vi "Set SG Path.vi"(0 "Path in":refnum<class "SA Path.lvclass">, 5 "Cal point in":T1, 11 "error in":errorcluster) -> (4 "Path out":refnum<class "SA Path.lvclass">, 6 "Cal point out":T1, 8 "Source Gain":dbl, 10 "Digital Gain":dbl, 15 "error out":errorcluster)   [LabVIEW 2023, in "RFFixtureCharact.PXI.lvlib" / "SA Path.lvclass"]
uses:
  SA Path.lvclass
  Public/Base Classes/Scalar/Scalar Path/Type Definitions/Cal Point.ctl
  <vilib>/addons/_RFCalAndCharactDatabase/NI_RFCalAndCharact_Database_API.lvlibp/Characterization/Controls/Type.ctl
  Public/Base Classes/Scalar/SA Abstract Path/SA Abstract Path.lvclass/SA Abstract Path.ctl
  Public/Base Classes/Scalar/SA Abstract Path/Properties/Read Cal Tone Pin.vi
  <instrlib>/niRFSG/niRFSG.llb/niRFSG Create De-embedding S-parameter Table (array).vi
  Public/Base Classes/Scalar/SA Path/SA Path.lvclass
  <vilib>/addons/_RFCalAndCharactDatabase/NI_RFCalAndCharact_Database_API.lvlibp/Characterization/Characterization.lvlib
  Public/Base Classes/Scalar/Scalar Path/Scalar Path.lvclass
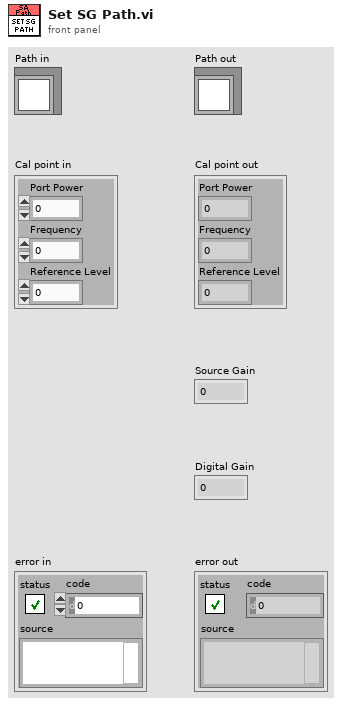
[diagram p1: front panel]
types:
  T1 = typedef "RFFixtureCharact.Public.lvlib/Scalar Path.lvclass/Cal Point.ctl" = cluster{"Port Power":dbl, "Frequency":dbl, "Reference Level":dbl}
  T2 = typedef "NI_RFCalAndCharact_Database_API.lvlibp/Characterization.lvlib/Type.ctl" = u16
  T3 = typedef "NI_RFCalAndCharact_Database_API.lvlibp/Characterization.lvlib/Path Handle.ctl" = refnum<k24>
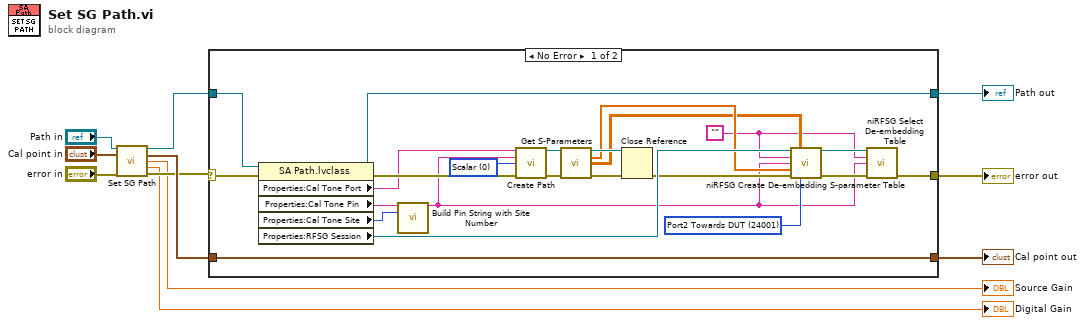
[diagram p0: block diagram]
diagram:
  n1 = call-parent "Set SG Path.vi"("Path in"="Path in", "Cal point in"="Cal point in", "error in (no error)"="error in") -> ("Path out"=w5:refnum<class "SA Path.lvclass">, "Cal point out"=w6:T1, "Source Gain"=→"Source Gain":dbl, "Digital Gain"=→"Digital Gain":dbl, "error out"=w3:errorcluster)  [unwired: 8 in]
  n2 = case shown="No Error" w3 {
    selector: w3 -> [w34 w37]
    tunnel: w5 -> [w33 w36]
    tunnel: [w32 w36] -> w10
    tunnel: [w17 w37] -> w9
    tunnel: [w13 w35] -> w11
    tunnel: w6 -> [w13 w35]
    frame No Error {
      w12 = ""
      w19 = 24001 items=["Port1 Towards DUT"=24000, "Port2 Towards DUT"=24001] ("S-parameters orientation")
      w30 = T2 0 items=["Scalar", "Vector"] ("Type")
      n3 = property class="SA Path.lvclass"(reference=w33, error in=w34) -> (reference out=w32:refnum<class "SA Path.lvclass">, error out=w27:errorcluster, "Properties:Cal Tone Port"=w15:string, "Properties:Cal Tone Pin"=w26:string, "Properties:Cal Tone Site"=w25:i32, "Properties:RFSG Session"=w31:refnum<k15>)
      n4 = call <vilib>:"Build Pin String with Site Number.vi"("Pin Name"=w26, "Site Number"=w25) -> ("Pin String"=w14:string)  [unwired: 13 in]
      n5 = call <vilib>:"Create Path.vi"("Port 1"=w15, "Port 2"=w14, "Type"=w30, "error in"=w27) -> ("Path"=w29:T3, "error out"=w28:errorcluster)  [unwired: 10 in]
      n6 = call <vilib>:"Get S-Parameters.vi"("Path In"=w29, "error in"=w28) -> ("Path Out"=w23:T3, "Frequencies (Hz)"=w21:dbl[], "S-Parameters"=w20:cdb[][][], "error out"=w24:errorcluster)  [unwired: 10 in]
      n7 = Close Reference(reference=w23, error in (no error)=w24) -> (error out=w22:errorcluster)
      n8 = call-poly <instrlib>:"niRFSG Create De-embedding S-parameter Table.vi"("instrument handle"=w31, "S-parameter table"=w20, "port"=w12, "table name"=w14, "frequencies"=w21, "error in"=w22, "S-parameters orientation"=w19) -> ("instrument handle out"=w16:refnum<k15>, "error out"=w18:errorcluster)  [unwired: 7 in]
      n9 = call <instrlib>:"niRFSG Select De-embedding Table.vi"("instrument handle"=w16, "port"=w12, "table name"=w14, "error in"=w18) -> ("error out"=w17:errorcluster)  [unwired: 10 in, 1 out]
    }
    frame Error {
    }
  }
  "error out" <- w9
  "Cal point out" <- w11
  "Path out" <- w10
